vi "Update X.vi"(8 "error in (no error)":errorcluster, 10 "SLAM In":T3, 11 "New LM's In":T2(array[cluster])) -> (0 "error out":errorcluster, 2 "SLAM Out":T3, 3 "New LM's Out":T2(array[cluster]))   [LabVIEW 2009]
uses:
  <vilib>/Analysis/Matrix/Datatypes/RealMatrix.ctl
  Controls/SLAM.ctl
  <vilib>/Analysis/baseanly.llb/Real A x B.vi
  <vilib>/Analysis/Matrix/NI_Matrix.lvlib
  <vilib>/Analysis/NI_AALBase.lvlib
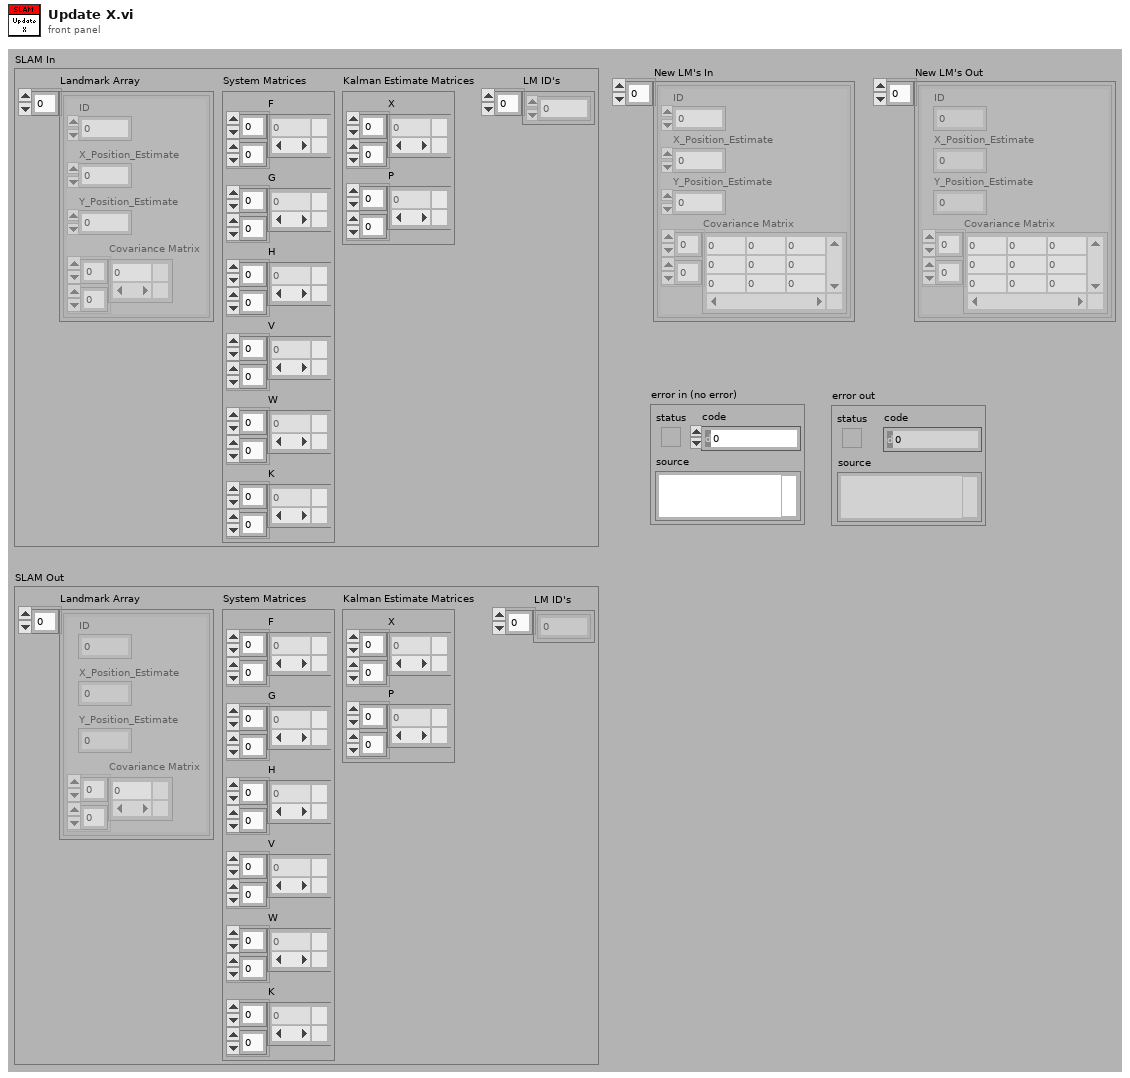
[diagram p1: front panel]
types:
  T1 = typedef "NI_Matrix.lvlib/RealMatrix.ctl" = dbl[][]
  T2 = cluster{"ID":dbl, "X_Position_Estimate":dbl, "Y_Position_Estimate":dbl, "Covariance Matrix":T1}[]
  T3 = typedef "SLAM.ctl" = cluster{"Landmark Array":cluster{"ID":dbl, "X_Position_Estimate":dbl, "Y_Position_Estimate":dbl, "Covariance Matrix":T1}[], "System Matrices":cluster{"F":T1, "G":T1, "H":T1, "V":T1, "W":T1, "K":T1}, "Kalman Estimate Matrices":cluster{"X":T1, "P":T1}, "LM ID's":dbl[]}
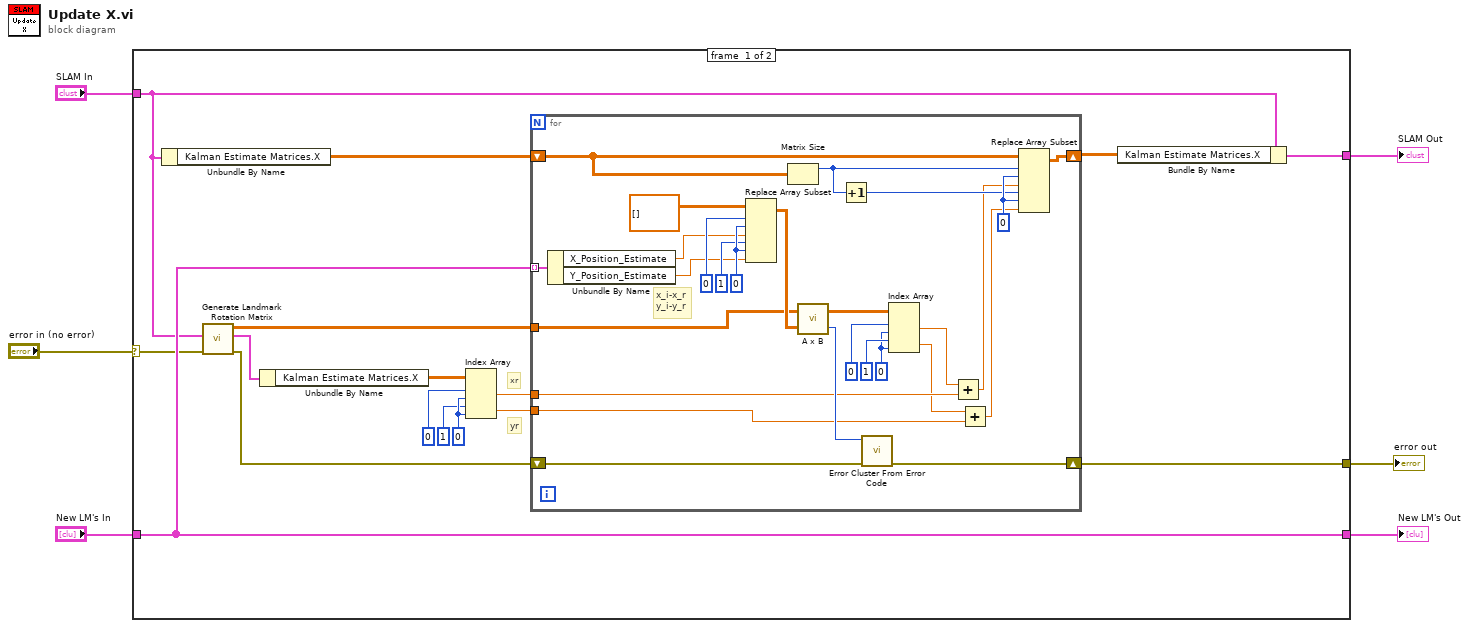
[diagram p0: block diagram]
diagram:
  n1 = case shown="No Error" "error in (no error)" {
    selector: "error in (no error)" -> [w9 w50]
    tunnel: "SLAM In" -> [w18 w51]
    tunnel: "New LM's In" -> [w19 w52]
    tunnel: [w22 w51] -> w4
    tunnel: [w19 w52] -> w3
    tunnel: [w7 w50] -> w1
    frame #0 {
      w14 = 0 ("index (col)")
      # "yr"
      # "xr"
      n2 = Unbundle By Name(w18) -> ("Kalman Estimate Matrices.X"=w20:T1)
      n3 = call "Generate Landmark Rotation Matrix.vi"("error in (no error)"=w9, "SLAM In"=w18) -> ("error out"=w8:errorcluster, "SLAM Out"=w16:T3, "Rotation matrix"=w17:T1)  [unwired: 7 in]
      n4 = Unbundle By Name(w16) -> ("Kalman Estimate Matrices.X"=w15:T1)
      n5 = Index Array(array=w15, index (row) #1=0 ("disabled index (row)"), index (col) #1=w14, index (row) #2=1 ("index (col)"), index (col) #2=w14) -> (element #1=w11:dbl, element #2=w10:dbl)
      n6 = for {
        shift-right: [w49] -> w21
        shift-left: w20 -> [w46]
        tunnel: w19 -> [w48] mode=indexing
        tunnel: w17 -> [w23]
        tunnel: w11 -> [w29]
        tunnel: w10 -> [w27]
        shift-right: [w35] -> w7
        shift-left: w8 -> [w37]
        w32 = 0 ("index (col)")
        w42 = 0 ("index (col)")
        w47 = 0 ("index (col)")
        # "x_i-x_r\ny_i-y_r"
        n7 = Unbundle By Name(w48) -> ("X_Position_Estimate"=w39:dbl, "Y_Position_Estimate"=w38:dbl)
        n8 = Replace Array Subset(array=T1 [] ("matrix"), new element #1=w39, index (row) #1=0 ("disabled index (row)"), index (col) #1=w42, new element #2=w38, index (row) #2=1 ("index (col)"), index (col) #2=w42) -> (w24:T1)
        n9 = Matrix Size(0:w46) -> (1:w45:i32)  [unwired: 1 out]
        n10 = call-poly <vilib>:"A x B.vi"("B"=w24, "A"=w23) -> ("error"=w36:i32, "A x B"=w31:T1)
        n11 = Increment(x=w45) -> (x+1=w44:i32)
        n12 = call <vilib>:"Error Cluster From Error Code.vi"("error in (no error)"=w37, "error code (0)"=w36) -> ("error out"=w35:errorcluster)  [unwired: 7 in]
        n13 = Index Array(array=w31, index (row) #1=0 ("disabled index (row)"), index (col) #1=w32, index (row) #2=1 ("index (col)"), index (col) #2=w32) -> (element #1=w30:dbl, element #2=w28:dbl)
        n14 = Add(x=w30, y=w29) -> (x+y=w26:dbl)
        n15 = Add(x=w28, y=w27) -> (x+y=w25:dbl)
        n16 = Replace Array Subset(array=w46, new element #1=w26, index (row) #1=w45, index (col) #1=w47, new element #2=w25, index (row) #2=w44, index (col) #2=w47) -> (w49:T1)
      }
      n17 = Bundle By Name(cluster=w18, "Kalman Estimate Matrices.X"=w21) -> (w22:T3)
    }
    frame #1 {
    }
  }
  "New LM's Out" <- w3
  "SLAM Out" <- w4
  "error out" <- w1
